vi "TSM Relay Configuration Publish Desired State.vi"(0 "TSM Relay Configuration in":T1 {"SSC Relay with Action"."Relay Action" items=["Open Relay"=20, "Close Relay"=21]}, 1 "Published Data Id":string, 7 "Completed Relay Operations":T4[](array[typedef]) {"Desired State" items=["Open Relay"=20, "Close Relay"=21]}, 11 "error in":errorcluster) -> (4 "TSM Relay Configuration out":T1 {"SSC Relay with Action"."Relay Action" items=["Open Relay"=20, "Close Relay"=21]}, 15 "error out":errorcluster)   [LabVIEW 2019]
doc: "This VI publishes the Desired State information from each Relay in the TSM Relay Configuration."
uses:
  SubVIs/TSM Relay Config.ctl
  <vilib>/NI_TestStand_SemiconductorModule/NI_TestStand_Semiconductor_Module.lvlibp/PinMap/PinQueryContext/MultiplePinMultipleSessionQueryContext/MultiplePinMultipleSessionQueryContext.lvclass
  C:/Program Files/National Instruments/LabVIEW 2019/vi.lib/NI_TestStand_SemiconductorModule/NI_TestStand_Semiconductor_Module.lvlibp/PinMap/PinQueryContext/MultipleSessionPinQueryContext.lvclass
  SSC/SSC Relay.ctl
  <instrlib>/niSwitch/niSwitch.llb/niSwitch Relay Action.ctl
  SubVIs/TSM Relay Completed Operations.ctl
  <vilib>/NI_TestStand_SemiconductorModule/NI_TestStand_Semiconductor_Module.lvlibp/PinMap/General/Publish/PublishDataDouble2D.vi
  <vilib>/NI_TestStand_SemiconductorModule/NI_TestStand_Semiconductor_Module.lvlibp
  C:/Program Files/National Instruments/LabVIEW 2019/vi.lib/NI_TestStand_SemiconductorModule/NI_TestStand_Semiconductor_Module.lvlibp/PinMap/PinQueryContext/PinQueryContext.lvclass
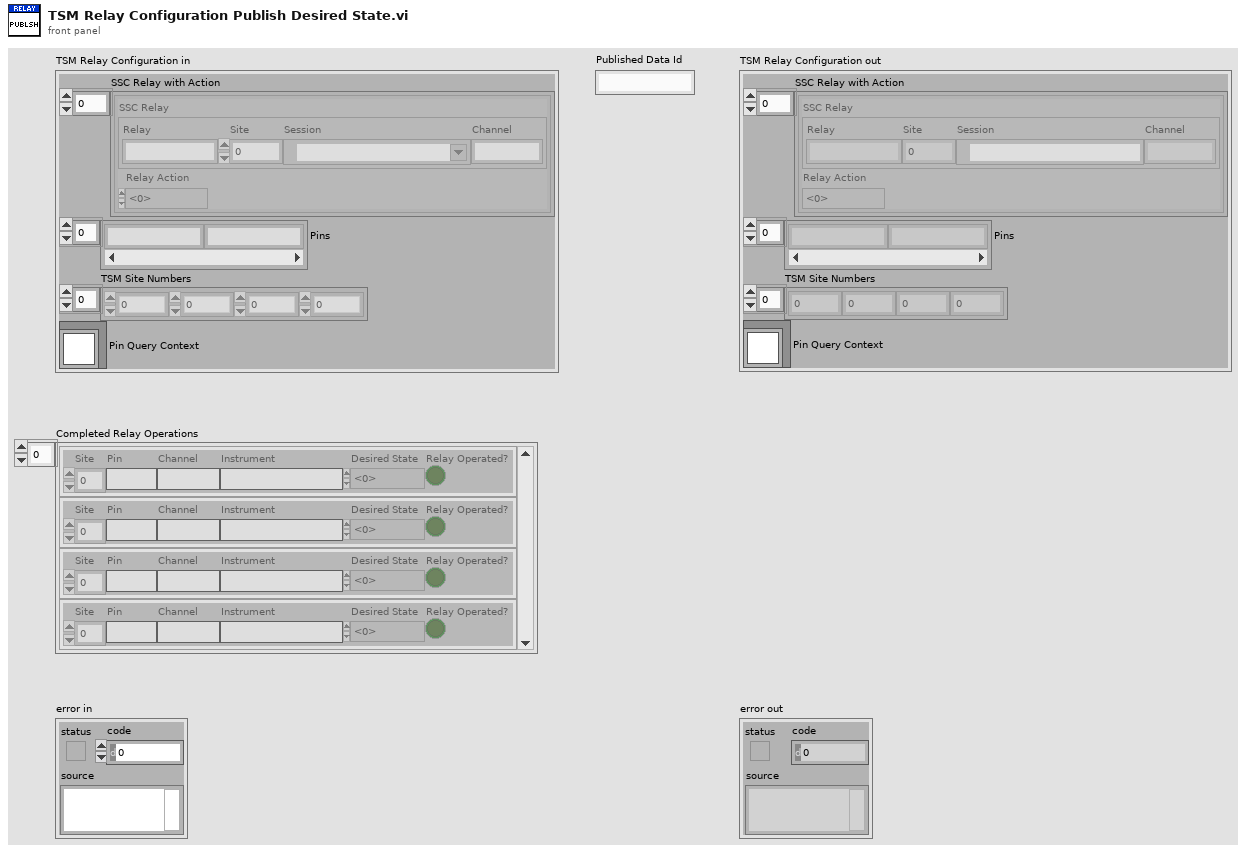
[diagram p1: front panel]
types:
  T1 = typedef "TSM Relay Config.ctl" = cluster{"SSC Relay with Action":cluster{"SSC Relay":T2, "Relay Action":T3}[], "Pins":string[], "TSM Site Numbers":i32[], "Pin Query Context":refnum<class "MultiplePinMultipleSessionQueryContext.lvclass">}
  T2 = typedef "SSC Relay.ctl" = cluster{"Relay":string, "Site":i32, "Session":refnum<k15>, "Channel":string}
  T3 = typedef "niSwitch Relay Action.ctl" = i32
  T4 = typedef "TSM Relay Completed Operations.ctl" = cluster{"Site":i32, "Pin":string, "Channel":string, "Instrument":string, "Desired State":T3, "Relay Operated?":bool}
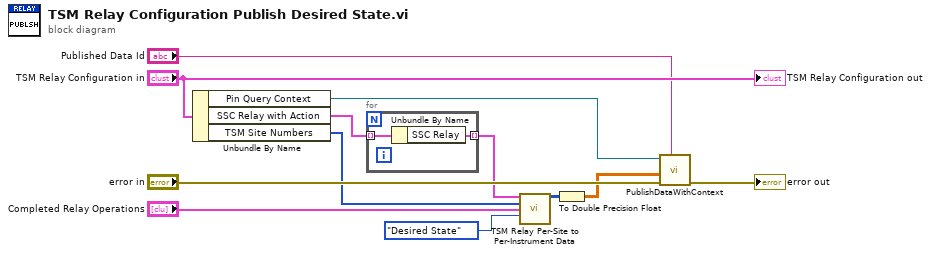
[diagram p0: block diagram]
diagram:
  n1 = Unbundle By Name("TSM Relay Configuration in") -> ("Pin Query Context"=w12:refnum<class "MultiplePinMultipleSessionQueryContext.lvclass">, "SSC Relay with Action"=w6:cluster{"SSC Relay":T2, "Relay Action":T3}[], "TSM Site Numbers"=w7:i32[])
  n2 = for {
    tunnel: w6 -> [w14] mode=indexing
    tunnel: [w13] -> w5 mode=indexing
    n3 = Unbundle By Name(w14) -> ("SSC Relay"=w13:T2)
  }
  n4 = call "TSM Relay Per-Site to Per-Instrument Data.vi"("SSC Relay"=w5, "TSM Site Numbers"=w7, "Completed Relay Operations"="Completed Relay Operations", "Selection"=enum16{"Desired State", "Relay Operated?"}."Desired State") -> ("Per-Instrument Per-Relay Data"=w1:i32[][])  [unwired: 11 in]
  n5 = To Double Precision Float(number=w1) -> (double precision float=w9:dbl[][])
  n6 = call-poly <vilib>:"PublishDataWithContext.vi"("Published Data Id"="Published Data Id", "error in (no error)"="error in", "Data In"=w9, "Pin Query Context"=w12) -> ("error out"=→"error out":errorcluster)  [unwired: 6 in, 1 out]
  "TSM Relay Configuration out" <- "TSM Relay Configuration in"
